vi "Convert SXM to PNG.vi"() -> ()   [LabVIEW 2019]
doc: "Converts Nanonis scan files (.sxm) into images (bmp or png). You can select multiple sxm files at once in the file dialog (use Shift or Ctrl).\n\n<B>Channel</B>: channel to export. If acquired, Z is always channel 0.\n<B>Scan direction</B>: direction to export.\n\n<B>Color type</B>: select between 8-bit greyscale (black to white) and 24-bit color (black to selected Color to white).\n<B>Color</B>: color for 24-bit color type.\n<B>Format</B>: select between bitmap (bmp) and portable network graphics (png).\n\n- Nanonis Programming Interface -"
uses:
  Instance           1 26Saved   Convert SXM to PNG .vi
  <userlib>/Nanonis Prog Interface V5/Nanonis Prog Interface.lvlib
panel:
  out "error out":errorcluster
  out "Output file":path
  out "Direction":string="Down"
  in  "Format":enum16{"bmp", "png"}(ring)=enum."png"
  in  "Color type":enum16{"8-bit greyscale", "24-bit color"}(ring)=enum."24-bit color"
  in  "Channel":i8 min=0
  in  "Scan direction":bool=TRUE
  in  "Color":u32(colorbox)=16731714
  out "Scan":picture
  # "Output"
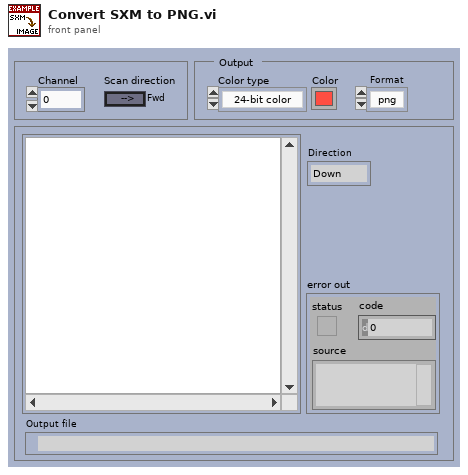
[diagram p1: front panel]
types:
  T1 = cluster{"up/down":bool, "time/line":sgl, "starttime":timestamp, "endtime":timestamp}
  T2 = typedef "imagedata.ctl" = cluster{"image type":i32, "image depth":i32, "image":u8[], "mask":u8[], "colors":u32[], "Rectangle":cluster{"left":i16, "top":i16, "right":i16, "bottom":i16}}
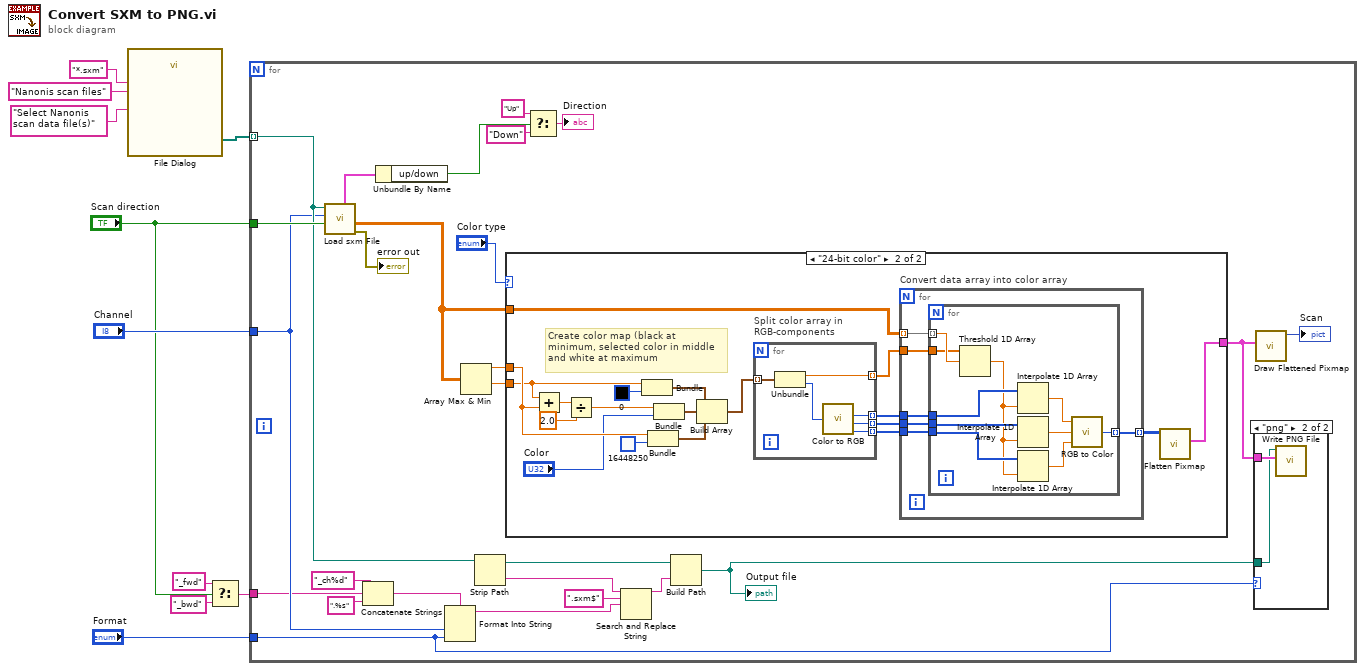
[diagram p0: block diagram]
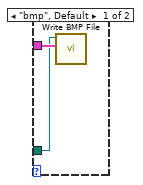
[diagram p2: hidden frame]
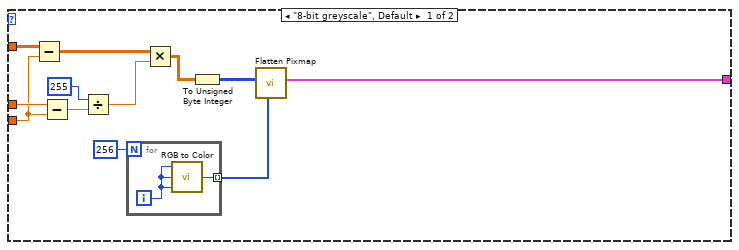
[diagram p3: hidden frame]
diagram:
  n1 = call "File Dialog"("prompt"="Select Nanonis scan data file(s)", "pattern (all files)"="*.sxm", "pattern label"="Nanonis scan files") -> ("selected paths"=w6:path[])  [unwired: 9 in, 3 out]
  n2 = Select(t="_fwd" ("pattern (all files)"), s="Scan direction", f="_bwd" ("pattern (all files)")) -> (s? t:f=w1:string)
  n3 = for {
    tunnel: "Channel" -> [w20]
    tunnel: "Scan direction" -> [w36]
    tunnel: w6 -> [w31] mode=indexing
    tunnel: "Format" -> [w21]
    tunnel: w1 -> [w15]
    n4 = call <userlib>:"Load sxm File.vi"("Scan direction"=w36, "Read channel"=w20, "Scan data file"=w31) -> ("error out"=→"error out":errorcluster, "Data"=w11:sgl[][], "Scan param"=w17:T1)  [unwired: 3 in, 3 out]
    n5 = Concatenate Strings("_ch%d" ("format string"), w15, ".%s" ("format string")) -> (w13:string)
    n6 = Unbundle By Name(w17) -> ("up/down"=w18:bool)
    n7 = Format Into String(format string=w13, w20, w21) -> (resulting string=w29:string)  [unwired: 2 in, 1 out]
    n8 = Array Max & Min(array=w11) -> (max value=w34:sgl, min value=w35:sgl)  [unwired: 2 out]
    n9 = Strip Path(path=w31) -> (stripped path=w26:path, name=w28:string)
    n10 = case shown="\"24-bit color\"" "Color type" {
      tunnel: w35 -> [w42 w57]
      tunnel: w34 -> [w45 w58]
      tunnel: w11 -> [w43 w68]
      tunnel: [w41 w67] -> w32
      frame "8-bit greyscale", Default {
        n11 = Subtract(x=w43, y=w42) -> (x-y=w46:sgl[][])
        n12 = Subtract(x=w45, y=w42) -> (x-y=w47:sgl)
        n13 = Divide(x=u8 255, y=w47) -> (x/y=w51:sgl)
        n14 = for {
          N: 256 -> [_]
          tunnel: [w53] -> w48 mode=indexing
          i -> [w54]
          n15 = call <vilib>:"RGB to Color.vi"("B"=w54, "G"=w54, "R"=w54) -> ("Color"=w53:u32)
        }
        n16 = Multiply(x=w46, y=w51) -> (x*y=w44:sgl[][])
        n17 = To Unsigned Byte Integer(number=w44) -> (unsigned 8bit integer=w50:u8[][])
        n18 = call <vilib>:"Flatten Pixmap.vi"("colors"=w48, "8-bit pixmap"=w50) -> ("image data"=w41:T2)  [unwired: 9 in]
      }
      frame "24-bit color" {
        # "Create color map (black at minimum, selected color in middle and white at maximum"
        n19 = Add(x=w57, y=w58) -> (x+y=w66:sgl)
        n20 = Divide(x=w66, y=2.0) -> (x/y=w63:dbl)
        n21 = Bundle(w57, u32 0) -> (w61:cluster{sgl, u32})  [unwired: 1 in]
        n22 = Bundle(w58, u32 16448250) -> (w59:cluster{sgl, u32})  [unwired: 1 in]
        n23 = Bundle(w63, "Color"="Color") -> (w60:cluster{dbl, "Color":u32})  [unwired: 1 in]
        n24 = Build Array(w61, w60, w59) -> (w55:cluster{dbl, "Color":u32}[])
        n25 = for "Split color array in\nRGB-components" {
          tunnel: w55 -> [w95] mode=indexing
          tunnel: [w94] -> w69 mode=indexing
          tunnel: [w92] -> w70 mode=indexing
          tunnel: [w91] -> w71 mode=indexing
          tunnel: [w90] -> w72 mode=indexing
          n26 = Unbundle(w95) -> (w94:dbl, "Color"=w93:u32)
          n27 = call <vilib>:"Color to RGB.vi"("Color"=w93) -> ("R"=w92:u8, "G"=w91:u8, "B"=w90:u8)  [unwired: 1 out]
        }
        n28 = for "Convert data array into color array" {
          tunnel: w68 -> [w79] mode=indexing
          tunnel: w69 -> [w78]
          tunnel: w70 -> [w77]
          tunnel: w71 -> [w76]
          tunnel: w72 -> [w75]
          tunnel: [w74] -> w73 mode=indexing
          n29 = for {
            tunnel: w79 -> [w89] mode=indexing
            tunnel: w78 -> [w88]
            tunnel: w77 -> [w87]
            tunnel: w76 -> [w86]
            tunnel: w75 -> [w85]
            tunnel: [w80] -> w74 mode=indexing
            n30 = Threshold 1D Array(2:w89, 3:w88) -> (0:w84:dbl)  [unwired: 1 in]
            n31 = Interpolate 1D Array(1:w84, 2:w87) -> (0:w83:dbl)
            n32 = Interpolate 1D Array(1:w84, 2:w86) -> (0:w82:dbl)
            n33 = Interpolate 1D Array(1:w84, 2:w85) -> (0:w81:dbl)
            n34 = call <vilib>:"RGB to Color.vi"("B"=w81, "G"=w82, "R"=w83) -> ("Color"=w80:u32)
          }
        }
        n35 = call <vilib>:"Flatten Pixmap.vi"("24-bit pixmap"=w73) -> ("image data"=w67:T2)  [unwired: 10 in]
      }
    }
    n36 = Select(t="Up" ("pattern (all files)"), s=w18, f="Down" ("pattern (all files)")) -> (s? t:f=→"Direction":string)
    n37 = Search and Replace String(input string=w28, search string=".sxm$", replace string=w29) -> (result string=w27:string)  [unwired: 5 in, 3 out]
    n38 = Build Path(base path=w26, name or relative path=w27) -> (appended path=w22:path)
    "Output file" <- w22
    n39 = case shown="\"png\"" w21 {
      tunnel: w32 -> [w38 w40]
      tunnel: w22 -> [w37 w39]
      frame "bmp", Default {
        n40 = call <vilib>:"Write BMP File.vi"("image data"=w38, "path to BMP file"=w37) -> ()  [unwired: 8 in, 2 out]
      }
      frame "png" {
        n41 = call <vilib>:"Write PNG File.vi"("image data"=w40, "path to PNG file"=w39) -> ()  [unwired: 8 in, 2 out]
      }
    }
    n42 = call <vilib>:"Draw Flattened Pixmap.vi"("image data"=w32) -> ("new picture"=→"Scan":picture)  [unwired: 8 in]
  }
